vi "SRV_Manage Loop Errors.vi"(6 "Loop Identifier":string, 7 "Clear Error? (T)":bool=TRUE, 8 "error in (no error)":errorcluster, 9 "Delay (1000 ms)":u32=1000) -> (0 "error out":errorcluster)   [LabVIEW 2014]
uses:
  <vilib>/Utility/error.llb/DialogType.ctl
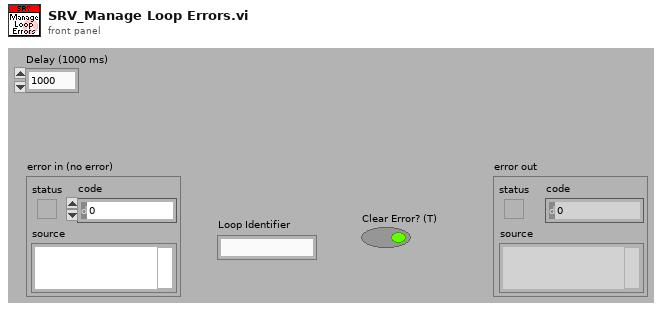
[diagram p1: front panel]
types:
  T1 = typedef "DialogType.ctl" = u16
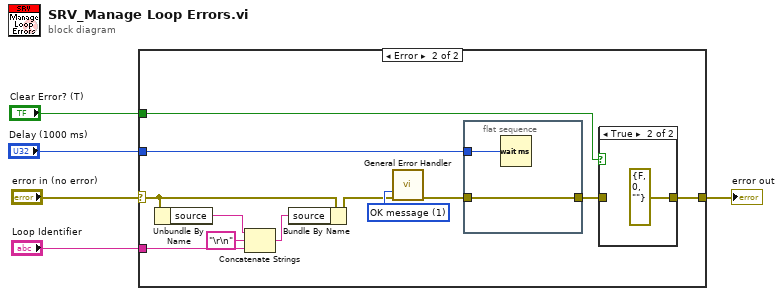
[diagram p0: block diagram]
diagram:
  n1 = case shown="Error" "error in (no error)" {
    selector: "error in (no error)" -> [w6 w14]
    tunnel: [w6 w7] -> w5
    tunnel: "Loop Identifier" -> [_ w15]
    tunnel: "Delay (1000 ms)" -> [_ w10]
    tunnel: "Clear Error? (T)" -> [_ w8]
    frame No Error {
    }
    frame Error {
      w18 = T1 1 items=["no dialog", "OK message", "continue or stop message", "OK message + warnings", "continue/stop + warnings"] ("type of dialog (OK msg:1)")
      n2 = Unbundle By Name(w14) -> ("source"=w17:string)
      n3 = Concatenate Strings(w17, "\r\n" ("string"), w15) -> (w12:string)
      n4 = Bundle By Name(cluster=w14, "source"=w12) -> (w13:errorcluster)
      n5 = call <vilib>:"General Error Handler.vi"("type of dialog (OK msg:1)"=w18, "error in (no error)"=w13) -> ("error out"=w11:errorcluster)  [unwired: 9 in, 4 out]
      n6 = flat-sequence {
        tunnel: w11 -> [w21]
        tunnel: w10 -> [w22]
        tunnel: [w21] -> w9
        frame #0 {
          n7 = Wait (ms)(milliseconds to wait=w22) -> ()  [unwired: 1 out]
        }
      }
      n8 = case shown="True" w8 {
        tunnel: w9 -> [w19 _]
        tunnel: [w19 errorcluster {"status"=FALSE, "code"=0, "source"=""} ("error out")] -> w7
        frame False {
        }
        frame True {
        }
      }
    }
  }
  "error out" <- w5
